vi "Filter Wheel Control.vi"(7 "Calling VI Ref":refnum<vi>) -> ()   [LabVIEW 2020]
uses:
  <vilib>/Utility/miscctls.llb/LVPointTypeDef.ctl
  Hardware Configuration/Hardware Configuration Controls/Device Type.ctl
  Hardware Configuration/Hardware Configuration Controls/Device Function.ctl
  Filter Wheel Type Defs/Filter Wheel Names.ctl
  Device Library/Filter Wheels/FW Type Defs/FW Actions.ctl
panel:
  in  "Tab Control":enum32{"Wheel Control", "Setup"}(tab)
  in  "Filter Wheel":u16(ring) items=["Camera 2 Filter Wheel"]
  in  "Position":T1(radio)
  in  "Pos_Name_06":string
  in  "Pos_Name_07":string
  in  "Pos_Name_08":string
  in  "Pos_Name_09":string
  in  "Pos_Name_10":string
  in  "Filter_Wheel_Name":string
  in  "Pos_Name_01":string
  in  "Pos_Name_02":string
  in  "Pos_Name_03":string
  in  "Pos_Name_04":string
  in  "Pos_Name_05":string
  in  "Filter Wheel Setup":bool=TRUE
  in  "Quit":bool
  # "Filter Wheel Name:"
  # "Position 01 Name:"
  # "Position 06 Name:"
  # "Position 02 Name:"
  # "Position 07 Name:"
  # "Position 03 Name:"
  # "Position 08 Name:"
  # "Position 04 Name:"
  # "Position 09 Name:"
  # "Position 05 Name:"
  # "Position 10 Name:"
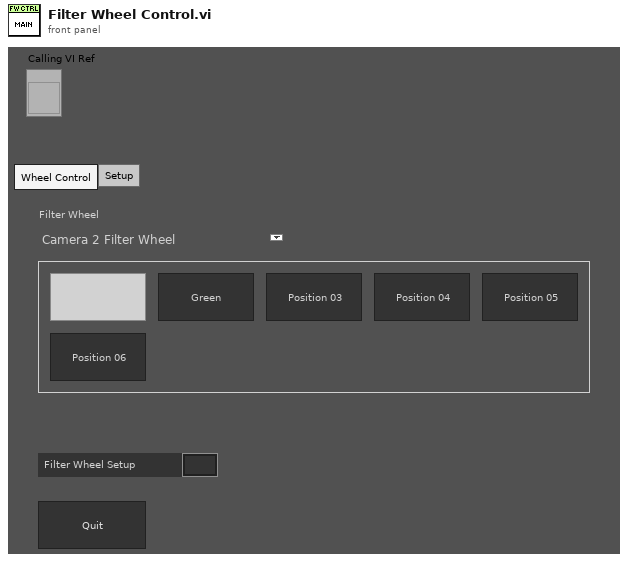
[diagram p1: front panel]
types:
  T1 = enum32{"Pos 01", "Pos 02", "Pos 03", "Pos 04", "Pos 05", "Pos 06", "Pos 07", "Pos 08", "Pos 09", "Pos 10"}
  T2 = typedef "FW Actions.ctl" = enum16{"Set Position", "Get Position", "Get Num Positions", "Set Speed", "Quit"}
  T3 = typedef "Filter Wheel Names.ctl" = string[][]
  T4 = typedef "Device Type.ctl" = enum16{"AOTF", "Camera", "Deformable Mirror", "Laser", "Shutter", "Stage", "Waveform", "FPGA", "Email", "Filter Wheel"}
  T5 = typedef "Device Function.ctl" = enum16{"Primary", "Secondary", "Overview", "Wide Field Drift Correction", "642 nm Excitation", "560 nm Excitation", "940 nm Excitation", "546 nm Excitation", "488 nm Excitation", "405 nm Excitation", "Objective Drift Correction", "4Pi Objective Lock", "Objective XY", "Objective Z", "Sample XY", "Sample Coarse Z", "Sample Z", "4Pi Lower", "4Pi Upper", "Mojo", "Adj Cavity", "Line Scanning", "Alert"}
  T6 = enum16{"Always On", "Always Off", "Off While Running"}
  T7 = typedef "LVPointTypeDef.ctl" = cluster{"Horizontal":i16, "Vertical":i16}
  T8 = enum8{"Enabled", "Disabled", "Disabled and Grayed Out"}
  T9 = typedef "LVRectTypeDef.ctl" = cluster{"Left":i16, "Top":i16, "Right":i16, "Bottom":i16}
  T10 = typedef "LVBoundsTypeDef.ctl" = cluster{"Width":u32, "Height":u32}
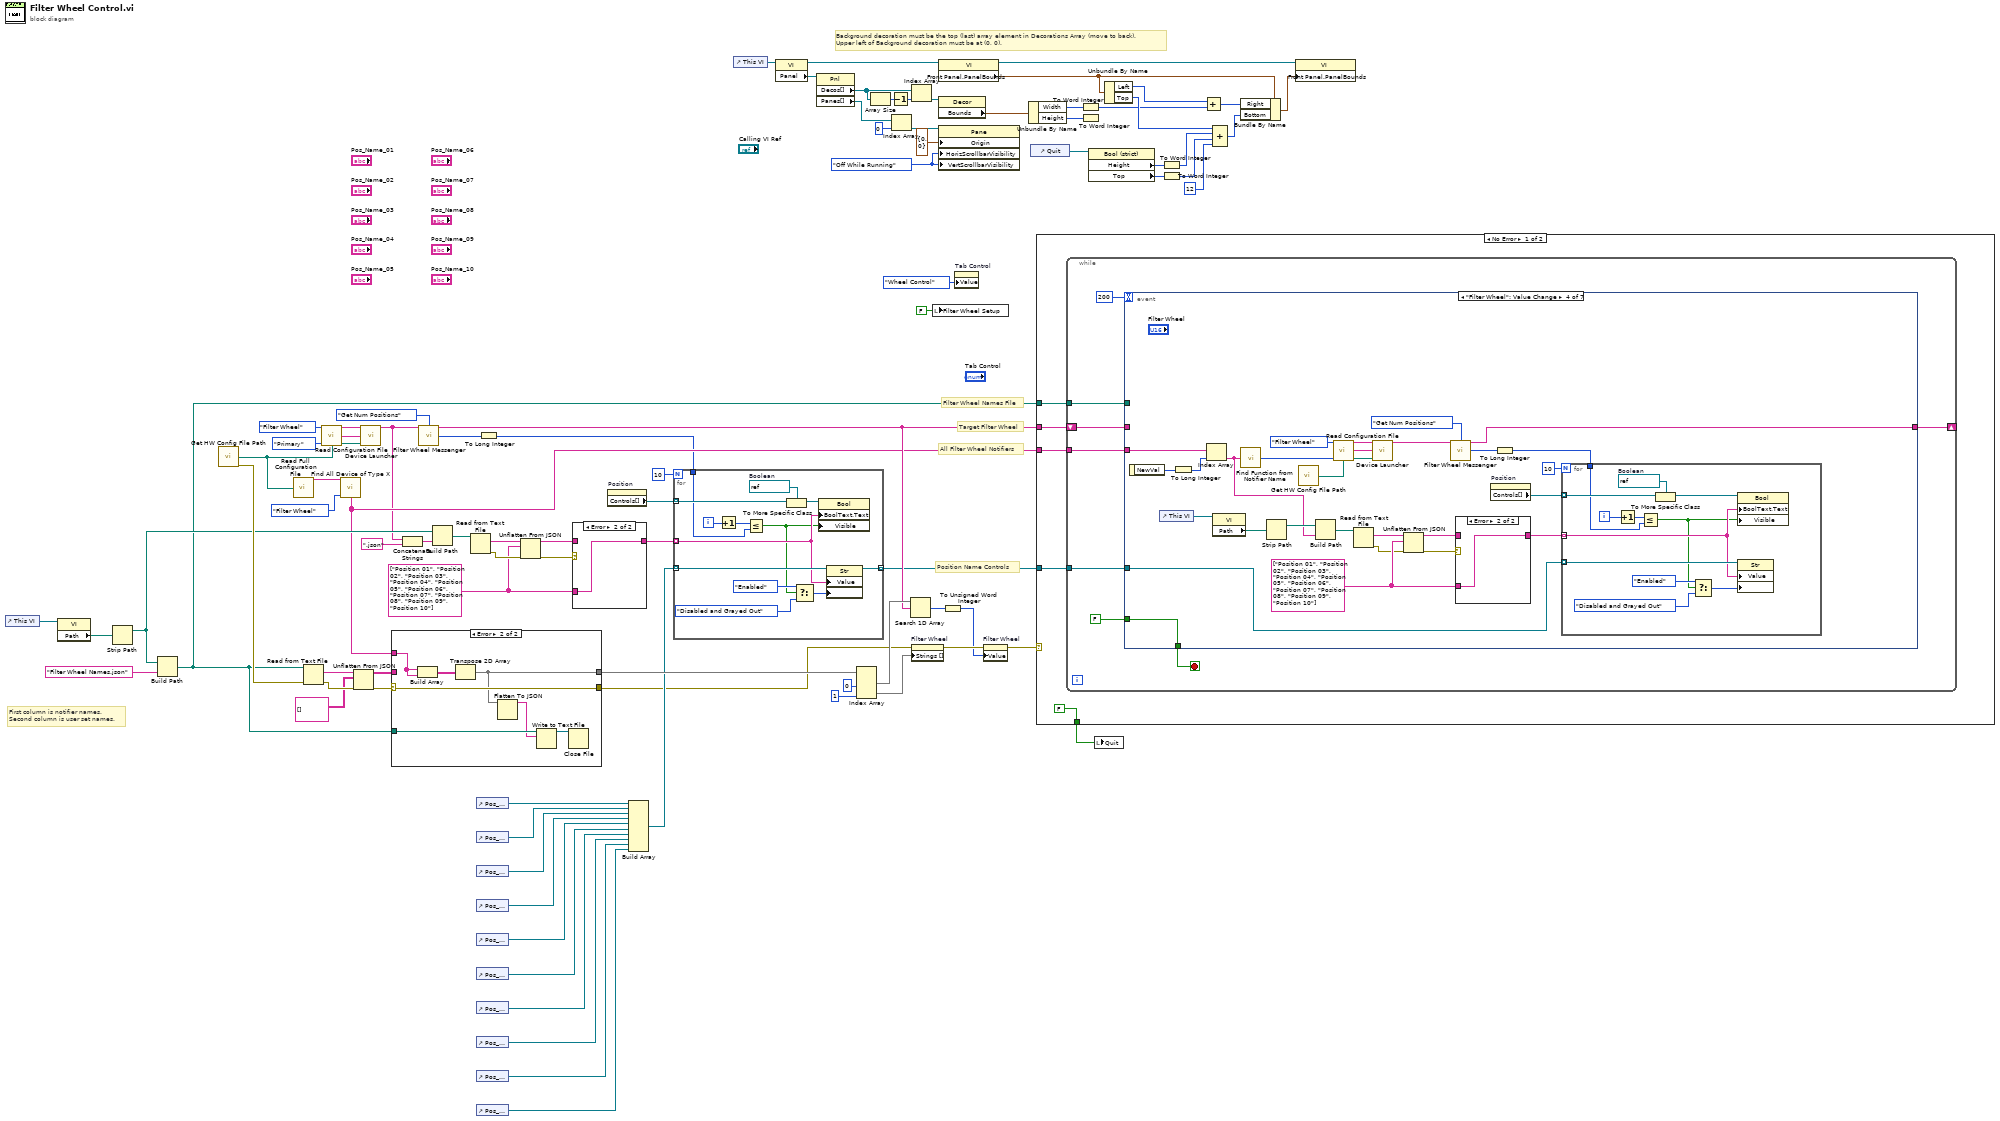
[diagram p0: block diagram]
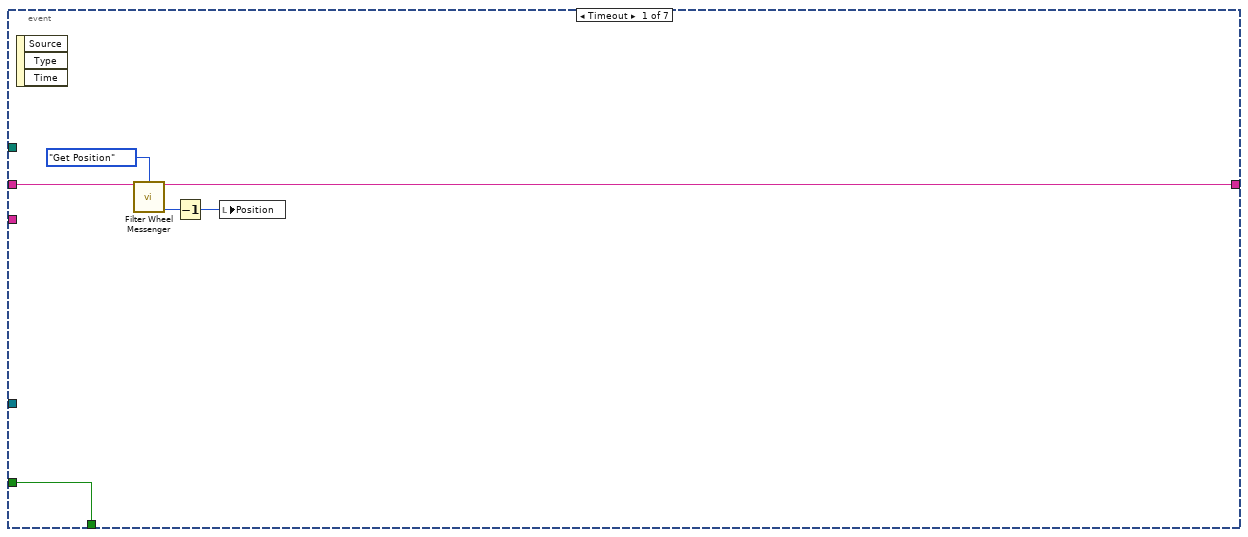
[diagram p2: hidden frame]
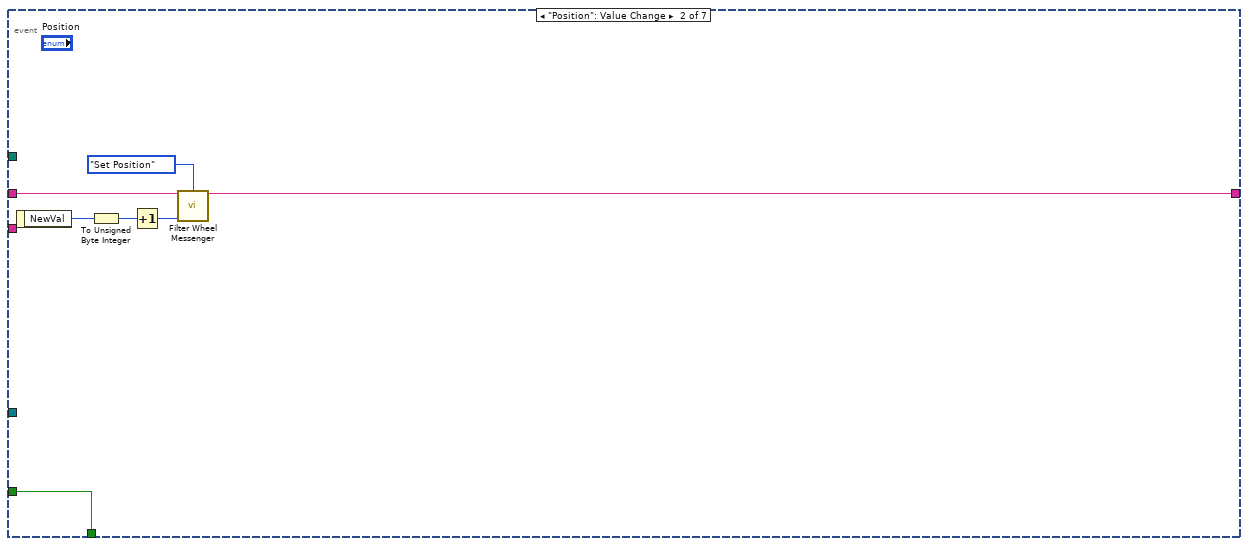
[diagram p3: hidden frame]
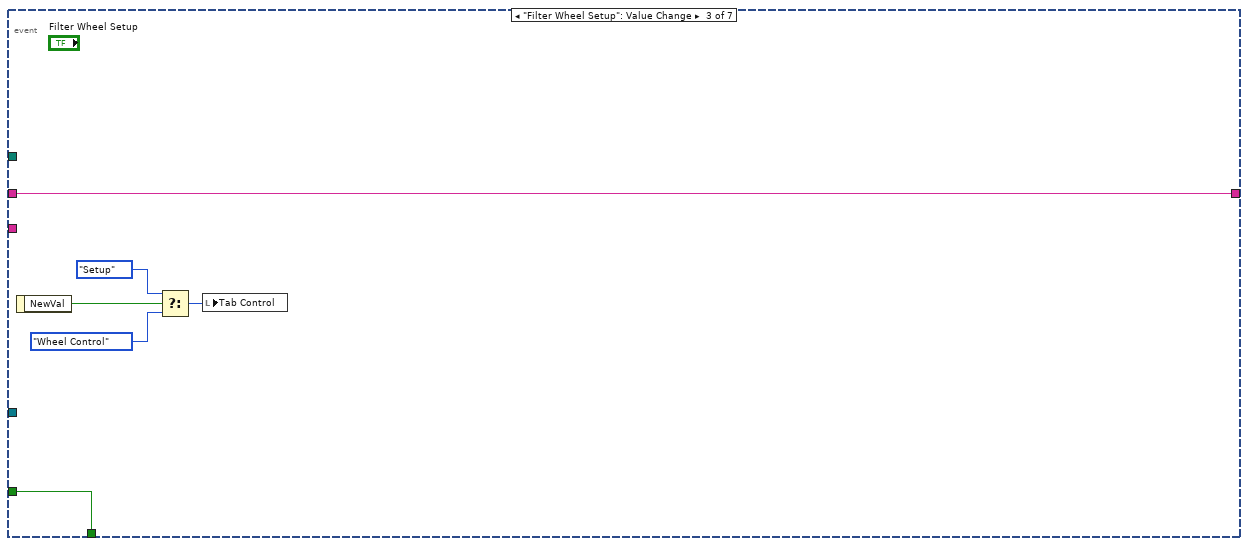
[diagram p4: hidden frame]
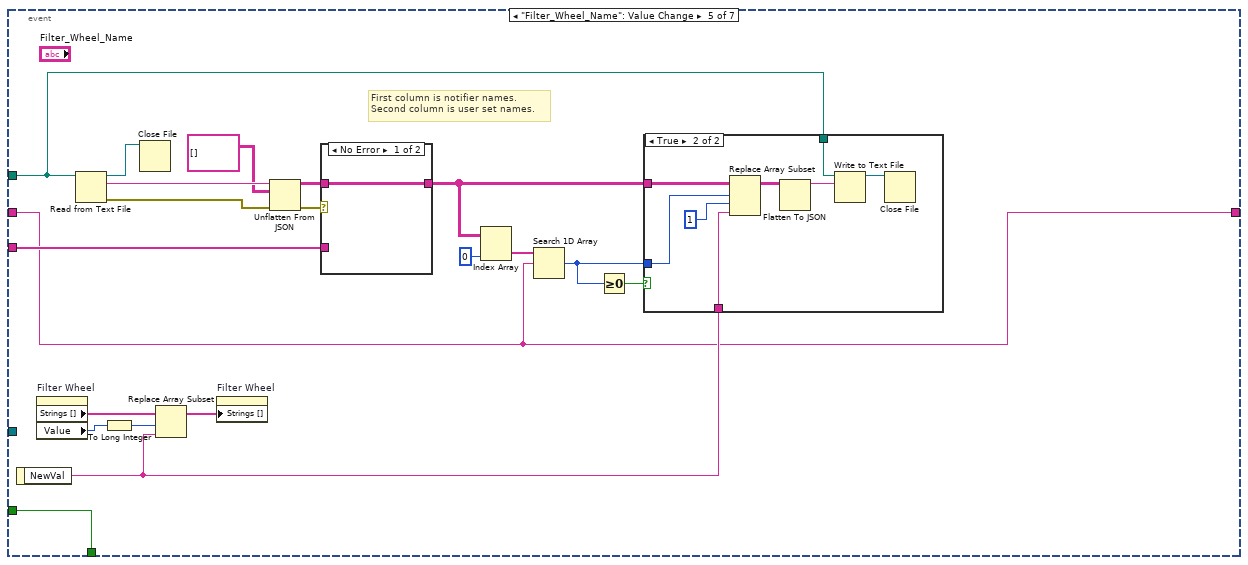
[diagram p6: hidden frame]
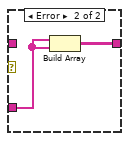
[diagram p8: hidden frame]
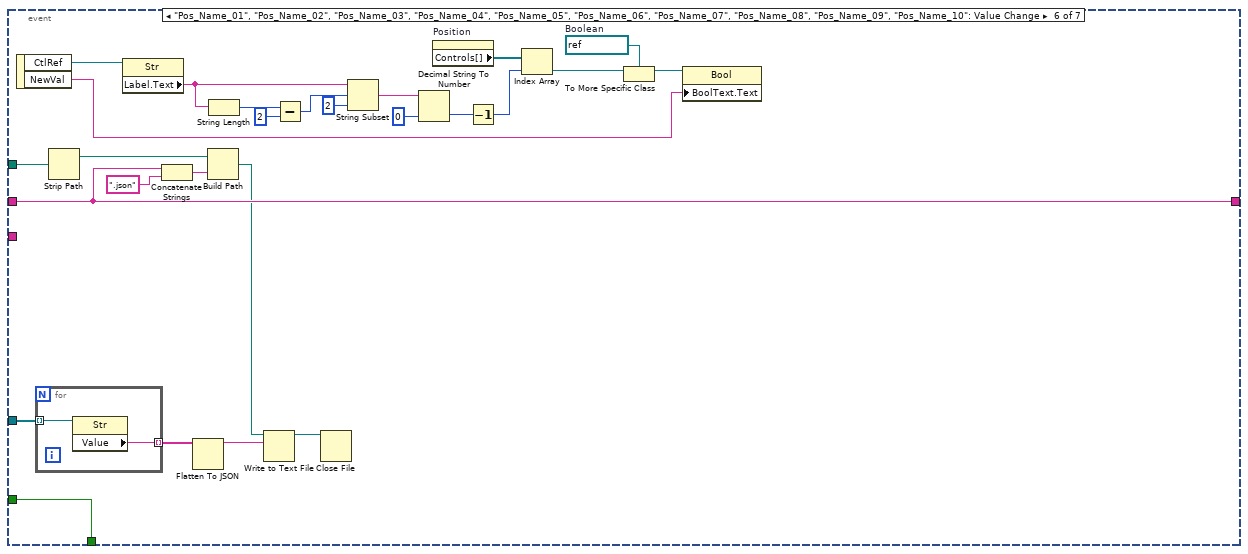
[diagram p9: hidden frame]
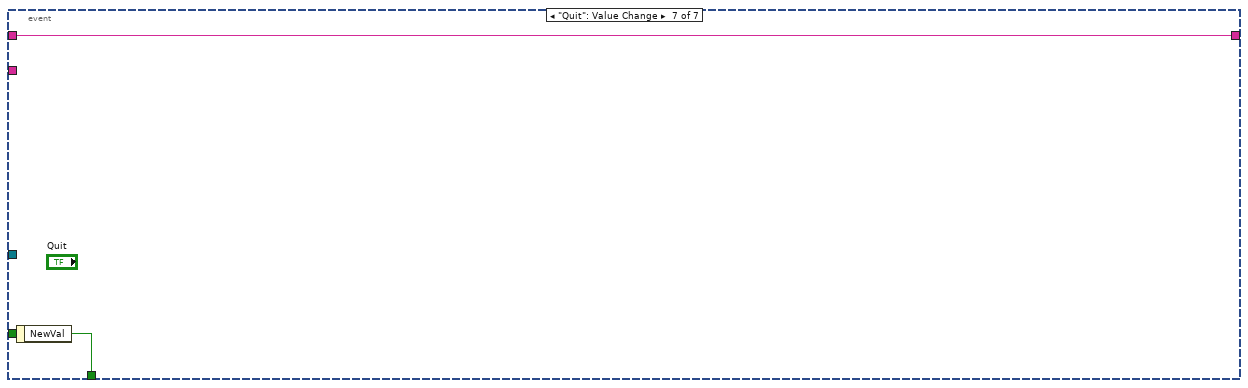
[diagram p10: hidden frame]
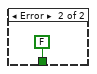
[diagram p11: hidden frame]
diagram:
  w18 = string[] ["Position 01", "Position 02", "Position 03", "Position 04", "Position 05", "Position 06", "Position 07", "Position 08", "Position 09", "Position 10"]
  w73 = T6."Off While Running" ("Vertical Scrollbar Visibility")
  # "Position Name Controls"
  # "All Filter Wheel Notifiers"
  # "Target Filter Wheel"
  # "Filter Wheel Names File"
  # "First column is notifier names.\nSecond column is user set names."
  # "Background decoration must be the top (last) array element in Decorations Array (move to back).\nUpper left of Background decoration must be at (0, 0)."
  n1 = control-ref of="This VI"() -> (w53:refnum<vi>)
  n2 = property class="VI"(reference=w53) -> ("Path"=w52:path)  [unwired: 1 in, 2 out]
  n3 = Strip Path(path=w52) -> (stripped path=w36:path)  [unwired: 1 out]
  n4 = Build Path(base path=w36, name or relative path="Filter Wheel Names.json") -> (appended path=w7:path)
  n5 = call "Get HW Config File Path.vi"() -> ("File Path"=w54:path, "Error"=w37:errorcluster)  [unwired: 14 in]
  n6 = call "Read Full Configuration File.vi"("Config File Path"=w54) -> ("Unique Notifier Names"=w56:string[])  [unwired: 11 in, 3 out]
  n7 = Read from Text File(file (use dialog)=w7, error in=w37) -> (text=w50:string, error out=w49:errorcluster)  [unwired: 2 in, 2 out]
  n8 = call "Read Configuration File.vi"("Device Type"=Device_Type."Filter Wheel", "Device Function"=Device_Function."Primary", "Config File Path"=w54) -> ("Unique Notifier Name"=w61:string, "Device Ports/IDs/Channels"=w59:string[], "Device Engine Path"=w60:path)  [unwired: 9 in, 1 out]
  n9 = call "Find All Device of Type X.vi"("Unique Notifier Names"=w56, "Device Type"=Device_Type."Filter Wheel") -> ("All Devices"=w10:string[])  [unwired: 12 in, 1 out]
  n10 = Unflatten From JSON(JSON string=w50, type and defaults=T3 [] ("Wheel Names"), error in (no error)=w49) -> (value=w46:T3, error out=w47:errorcluster)  [unwired: 4 in]
  n11 = call "Device Launcher.vi"("Notifier Name"=w61, "Device Ports/IDs/Channels"=w59, "Device Engine Path"=w60) -> ("Notifier Name"=w2:string)  [unwired: 11 in, 1 out]
  n12 = case shown="Error" w47 {
    selector: w47 -> [w91 w98]
    tunnel: w46 -> [w92 _]
    tunnel: [w92 w94] -> w45
    tunnel: w10 -> [_ w99]
    tunnel: [w91 w98] -> w12
    tunnel: w7 -> [_ w97]
    frame No Error {
    }
    frame Error {
      n13 = Build Array(w99, w99) -> (w95:string[][])
      n14 = Transpose 2D Array(2D array=w95) -> (transposed array=w94:string[][])
      n15 = Flatten To JSON(anything=w94) -> (JSON string=w93:string)  [unwired: 2 in, 1 out]
      n16 = Write to Text File(file (use dialog)=w97, text=w93) -> (refnum out=w96:refnum<file>)  [unwired: 2 in, 2 out]
      n17 = Close File(refnum=w96) -> ()  [unwired: 1 in, 2 out]
    }
  }
  n18 = Concatenate Strings(w2, ".json" ("string")) -> (w3:string)
  n19 = call "Filter Wheel Messenger.vi"("FW Notifier"=w2, "Actions"=FW_Actions."Get Num Positions") -> ("FW Notifier (Dup)"=w21:string, "Num Positions"=w9:u8)  [unwired: 11 in, 1 out]
  n20 = Build Path(base path=w36, name or relative path=w3) -> (appended path=w33:path)
  n21 = Read from Text File(file (use dialog)=w33) -> (text=w34:string, error out=w35:errorcluster)  [unwired: 3 in, 2 out]
  n22 = control-ref of="Pos_Name_01"() -> (w32:refnum<vi>)
  n23 = control-ref of="Pos_Name_02"() -> (w23:refnum<vi>)
  n24 = control-ref of="Pos_Name_03"() -> (w24:refnum<vi>)
  n25 = control-ref of="Pos_Name_04"() -> (w25:refnum<vi>)
  n26 = control-ref of="Pos_Name_05"() -> (w26:refnum<vi>)
  n27 = control-ref of="Pos_Name_06"() -> (w27:refnum<vi>)
  n28 = control-ref of="Pos_Name_07"() -> (w28:refnum<vi>)
  n29 = control-ref of="Pos_Name_08"() -> (w29:refnum<vi>)
  n30 = control-ref of="Pos_Name_09"() -> (w30:refnum<vi>)
  n31 = control-ref of="Pos_Name_10"() -> (w31:refnum<vi>)
  n32 = To Long Integer(number=w9) -> (32bit integer=w8:i32)
  n33 = Unflatten From JSON(JSON string=w34, type and defaults=w18, error in (no error)=w35) -> (value=w19:string[], error out=w20:errorcluster)  [unwired: 4 in]
  n34 = case shown="Error" w20 {
    tunnel: w19 -> [w100 _]
    tunnel: w18 -> [_ w101]
    tunnel: [w100 w101] -> w16
    frame No Error {
    }
    frame Error {
    }
  }
  n35 = property on="Position" class="RadioBtnsControl (strict)"() -> ("Controls[]"=w13:refnum<vi>[])  [unwired: 2 in, 2 out]
  n36 = Build Array(w32, w23, w24, w25, w26, w27, w28, w29, w30, w31) -> (w15:refnum<vi>[])
  n37 = for {
    N: 10 -> [_]
    tunnel: w16 -> [w109] mode=indexing
    tunnel: w15 -> [w114] mode=indexing
    tunnel: [w113] -> w14 mode=indexing
    tunnel: w13 -> [w112] mode=indexing
    tunnel: w8 -> [w106]
    i -> [w108]
    w111 = refnum<vi> refnum  # Boolean
    n38 = Increment(x=w108) -> (x+1=w107:i32)
    n39 = Less Or Equal?(x=w107, y=w106) -> (x <= y?=w102:bool)
    n40 = To More Specific Class(target class=w111, reference=w112) -> (specific class reference=w110:refnum<vi>)  [unwired: 1 in, 1 out]
    n41 = Select(t=T8."Enabled" ("Disabled"), s=w102, f=T8."Disabled and Grayed Out") -> (s? t:f=w104:T8)
    n42 = property class="Bool"(reference=w110, "BoolText.Text"=w109, "Visible"=w102) -> ()  [unwired: 1 in, 2 out]
    n43 = property class="Str"(reference=w114, "Value"=w109, "DisabledEnum"=w104) -> (reference out=w113:refnum<vi>)  [unwired: 1 in, 1 out]
  }
  n44 = control-ref of="This VI"() -> (w65:refnum<vi>)
  n45 = property class="VI"(reference=w65) -> (reference out=w74:refnum<vi>, "Panel"=w66:refnum<vi>)  [unwired: 1 in, 1 out]
  n46 = property class="Pnl"(reference=w66) -> ("Decos[]"=w64:refnum<vi>[], "Panes[]"=w70:refnum<vi>[])  [unwired: 1 in, 2 out]
  n47 = Index Array(array=w45, index (col) #1=0 ("disabled index (col)"), index (col) #2=1 ("index (col)")) -> (element #1=w38:string[], element #2=w39:string[])  [unwired: 2 in]
  n48 = Array Size(array=w64) -> (size(s)=w62:i32)
  n49 = Decrement(x=w62) -> (x-1=w63:i32)
  n50 = Index Array(array=w70, index=0) -> (element=w69:refnum<vi>)
  n51 = Search 1D Array(1D array=w38, element=w21) -> (index of element=w42:i32)  [unwired: 1 in]
  n52 = property on="Filter Wheel" class="Ring (strict)"(error in=w12, "Strings []"=w39) -> (error out=w43:errorcluster)  [unwired: 1 in, 1 out]
  n53 = Index Array(array=w64, index=w63) -> (element=w72:refnum<vi>)
  n54 = local write "Filter Wheel Setup"(FALSE ("Filter Wheel Setup")) -> ()
  n55 = property class="VI"(reference=w74) -> (reference out=w76:refnum<vi>, "Front Panel.PanelBounds"=w77:T9)  [unwired: 1 in, 1 out]
  n56 = property class="Decor"(reference=w72) -> ("Bounds"=w75:T10)  [unwired: 1 in, 2 out]
  n57 = property class="Pane"(reference=w69, "Origin"=T7 {"Horizontal"=0, "Vertical"=0}, "HorizScrollbarVisibility"=w73, "VertScrollbarVisibility"=w73) -> ()  [unwired: 1 in, 2 out]
  n58 = To Unsigned Word Integer(number=w42) -> (unsigned 16bit integer=w41:u16)
  n59 = property on="Tab Control" class="TabCtl (strict)"("Value"=enum32{"Wheel Control", "Setup"}."Wheel Control" ("Tab Control")) -> ()  [unwired: 2 in, 2 out]
  n60 = property on="Filter Wheel" class="Ring (strict)"(error in=w43, "Value"=w41) -> (error out=w11:errorcluster)  [unwired: 1 in, 1 out]
  n61 = Unbundle By Name(w75) -> ("Width"=w80:u32, "Height"=w83:u32)
  n62 = control-ref of="Quit"() -> (w67:refnum<vi>)
  n63 = case shown="No Error" w11 {
    tunnel: w7 -> [w119 _]
    tunnel: w21 -> [w118 _]
    tunnel: w14 -> [w117 _]
    tunnel: w10 -> [w116 _]
    tunnel: [FALSE FALSE] -> w4
    frame No Error {
      n64 = while {
        shift-right: [w121] -> _
        shift-left: w118 -> [w123]
        tunnel: w119 -> [w125]
        tunnel: w117 -> [w124]
        tunnel: w116 -> [w120]
        stop <- w126 stop-if-true
        n65 = event shown="[3] \"Filter Wheel\": Value Change" {
          selector: _ -> [_ _ _ _ _ _ _]
          dyn-events: _ -> [_ _ _ _ _ _ _]
          timeout: 200 -> [_ _ _ _ _ _ _]
          tunnel: FALSE -> [w133 w140 w146 w175 w209 w246 _]
          tunnel: [w133 w140 w146 w175 w209 w246 w250] -> w126
          tunnel: w125 -> [_ _ _ _ w190 w243 _]
          tunnel: w124 -> [_ _ _ w153 _ w245 _]
          tunnel: w123 -> [w130 w135 w141 _ w192 w240 w249]
          tunnel: [w129 w134 w141 w148 w192 w240 w249] -> w121
          tunnel: w120 -> [_ _ _ w174 w208 _ _]
          event Timeout {
            n66 = event-data() -> ()  [unwired: 1 in, 3 out]
            n67 = call "Filter Wheel Messenger.vi"("FW Notifier"=w130, "Actions"=FW_Actions."Get Position") -> ("FW Notifier (Dup)"=w129:string, "Current Position"=w131:u8)  [unwired: 11 in, 1 out]
            n68 = Decrement(x=w131) -> (x-1=w128:u8)
            n69 = local write "Position"(w128) -> ()
          }
          event "Position": Value Change {
            n70 = event-data() -> ("NewVal"=w139:T1)  [unwired: 1 in]
            n71 = To Unsigned Byte Integer(number=w139) -> (unsigned 8bit integer=w138:u8)
            n72 = Increment(x=w138) -> (x+1=w137:u8)
            n73 = call "Filter Wheel Messenger.vi"("FW Notifier"=w135, "Actions"=FW_Actions."Set Position", "Set Position"=w137) -> ("FW Notifier (Dup)"=w134:string)  [unwired: 10 in, 2 out]
          }
          event "Filter Wheel Setup": Value Change {
            n74 = event-data() -> ("NewVal"=w145:bool)  [unwired: 1 in]
            n75 = Select(t=enum32{"Wheel Control", "Setup"}."Setup" ("Tab Control"), s=w145, f=enum32{"Wheel Control", "Setup"}."Wheel Control" ("Tab Control")) -> (s? t:f=w142:enum32{"Wheel Control", "Setup"})
            n76 = local write "Tab Control"(w142) -> ()
          }
          event "Filter Wheel": Value Change {
            w163 = string[] ["Position 01", "Position 02", "Position 03", "Position 04", "Position 05", "Position 06", "Position 07", "Position 08", "Position 09", "Position 10"]
            n77 = event-data() -> ("NewVal"=w173:u16)  [unwired: 1 in]
            n78 = control-ref of="This VI"() -> (w157:refnum<vi>)
            n79 = To Long Integer(number=w173) -> (32bit integer=w172:i32)
            n80 = Index Array(array=w174, index=w172) -> (element=w154:string)
            n81 = property class="VI"(reference=w157) -> ("Path"=w156:path)  [unwired: 1 in, 2 out]
            n82 = call "Find Function from Notifier Name.vi"("Unique Notifier Name"=w154) -> ("Function"=w167:T5)  [unwired: 14 in]
            n83 = Strip Path(path=w156) -> (stripped path=w155:path)  [unwired: 1 out]
            n84 = call "Get HW Config File Path.vi"() -> ("File Path"=w147:path)  [unwired: 14 in, 1 out]
            n85 = Build Path(base path=w155, name or relative path=w154) -> (appended path=w160:path)
            n86 = call "Read Configuration File.vi"("Device Type"=Device_Type."Filter Wheel", "Device Function"=w167, "Config File Path"=w147) -> ("Unique Notifier Name"=w171:string, "Device Ports/IDs/Channels"=w169:string[], "Device Engine Path"=w170:path)  [unwired: 9 in, 1 out]
            n87 = Read from Text File(file (use dialog)=w160) -> (text=w159:string, error out=w158:errorcluster)  [unwired: 3 in, 2 out]
            n88 = call "Device Launcher.vi"("Notifier Name"=w171, "Device Ports/IDs/Channels"=w169, "Device Engine Path"=w170) -> ("Notifier Name"=w151:string)  [unwired: 11 in, 1 out]
            n89 = Unflatten From JSON(JSON string=w159, type and defaults=w163, error in (no error)=w158) -> (value=w162:string[], error out=w161:errorcluster)  [unwired: 4 in]
            n90 = call "Filter Wheel Messenger.vi"("FW Notifier"=w151, "Actions"=FW_Actions."Get Num Positions") -> ("FW Notifier (Dup)"=w148:string, "Num Positions"=w150:u8)  [unwired: 11 in, 1 out]
            n91 = case shown="Error" w161 {
              tunnel: w162 -> [w188 _]
              tunnel: w163 -> [_ w189]
              tunnel: [w188 w189] -> w165
              frame No Error {
              }
              frame Error {
              }
            }
            n92 = property on="Position" class="RadioBtnsControl (strict)"() -> ("Controls[]"=w166:refnum<vi>[])  [unwired: 2 in, 2 out]
            n93 = To Long Integer(number=w150) -> (32bit integer=w149:i32)
            n94 = for {
              N: 10 -> [_]
              tunnel: w165 -> [w183] mode=indexing
              tunnel: w153 -> [w187] mode=indexing
              tunnel: w166 -> [w186] mode=indexing
              tunnel: w149 -> [w180]
              i -> [w181]
              w185 = refnum<vi> refnum  # Boolean
              n95 = Increment(x=w181) -> (x+1=w182:i32)
              n96 = Less Or Equal?(x=w182, y=w180) -> (x <= y?=w176:bool)
              n97 = To More Specific Class(target class=w185, reference=w186) -> (specific class reference=w184:refnum<vi>)  [unwired: 1 in, 1 out]
              n98 = Select(t=T8."Enabled" ("Disabled"), s=w176, f=T8."Disabled and Grayed Out") -> (s? t:f=w177:T8)
              n99 = property class="Bool"(reference=w184, "BoolText.Text"=w183, "Visible"=w176) -> ()  [unwired: 1 in, 2 out]
              n100 = property class="Str"(reference=w187, "Value"=w183, "DisabledEnum"=w177) -> ()  [unwired: 1 in, 2 out]
            }
          }
          event "Filter_Wheel_Name": Value Change {
            # "First column is notifier names.\nSecond column is user set names."
            n101 = event-data() -> ("NewVal"=w193:string)  [unwired: 1 in]
            n102 = property on="Filter Wheel" class="Ring (strict)"() -> ("Strings []"=w202:string[], "Value"=w201:u16)  [unwired: 2 in, 2 out]
            n103 = Read from Text File(file (use dialog)=w190) -> (refnum out=w191:refnum<file>, text=w207:string, error out=w206:errorcluster)  [unwired: 3 in, 1 out]
            n104 = To Long Integer(number=w201) -> (32bit integer=w200:i32)
            n105 = Close File(refnum=w191) -> ()  [unwired: 1 in, 2 out]
            n106 = Replace Array Subset(array=w202, new element=w193, index=w200) -> (w199:string[])
            n107 = property on="Filter Wheel" class="Ring (strict)"("Strings []"=w199) -> ()  [unwired: 2 in, 2 out]
            n108 = Unflatten From JSON(JSON string=w207, type and defaults=T3 [] ("Wheel Names"), error in (no error)=w206) -> (value=w203:T3, error out=w204:errorcluster)  [unwired: 4 in]
            n109 = case shown="No Error" w204 {
              tunnel: [w218 w219] -> w198
              tunnel: w208 -> [_ w220]
              tunnel: w203 -> [w218 _]
              frame No Error {
              }
              frame Error {
                n110 = Build Array(w220, w220) -> (w219:string[][])
              }
            }
            n111 = Index Array(array=w198, index (col)=0 ("disabled index (col)")) -> (element=w196:string[])  [unwired: 1 in]
            n112 = Search 1D Array(1D array=w196, element=w192) -> (index of element=w194:i32)  [unwired: 1 in]
            n113 = Greater Or Equal To 0?(x=w194) -> (x >= 0?=w195:bool)
            n114 = case shown="True" w195 {
              tunnel: w198 -> [_ w216]
              tunnel: w194 -> [_ w215]
              tunnel: w193 -> [_ w214]
              tunnel: w190 -> [_ w210]
              frame False {
              }
              frame True {
                n115 = Replace Array Subset(array=w216, new element=w214, index (row)=w215, index (col)=1 ("disabled index (col)")) -> (w211:T3)
                n116 = Flatten To JSON(anything=w211) -> (JSON string=w213:string)  [unwired: 2 in, 1 out]
                n117 = Write to Text File(file (use dialog)=w210, text=w213) -> (refnum out=w212:refnum<file>)  [unwired: 2 in, 2 out]
                n118 = Close File(refnum=w212) -> ()  [unwired: 1 in, 2 out]
              }
            }
          }
          event "Pos_Name_01", "Pos_Name_02", "Pos_Name_03", "Pos_Name_04", "Pos_Name_05", "Pos_Name_06", "Pos_Name_07", "Pos_Name_08", "Pos_Name_09", "Pos_Name_10": Value Change {
            w236 = refnum<vi> refnum  # Boolean
            n119 = event-data() -> ("CtlRef"=w235:refnum<vi>, "NewVal"=w223:string)  [unwired: 1 in]
            n120 = for {
              tunnel: w245 -> [w248] mode=indexing
              tunnel: [w247] -> w244 mode=indexing
              n121 = property class="Str"(reference=w248) -> ("Value"=w247:string)  [unwired: 1 in, 2 out]
            }
            n122 = Strip Path(path=w243) -> (stripped path=w242:path)  [unwired: 1 out]
            n123 = property class="Str"(reference=w235) -> ("Label.Text"=w233:string)  [unwired: 1 in, 2 out]
            n124 = Concatenate Strings(w240, ".json" ("string")) -> (w241:string)
            n125 = Flatten To JSON(anything=w244) -> (JSON string=w238:string)  [unwired: 2 in, 1 out]
            n126 = Build Path(base path=w242, name or relative path=w241) -> (appended path=w237:path)
            n127 = String Length(string=w233) -> (length=w232:i32)
            n128 = Write to Text File(file (use dialog)=w237, text=w238) -> (refnum out=w222:refnum<file>)  [unwired: 2 in, 2 out]
            n129 = Subtract(x=w232, y=2) -> (x-y=w230:i32)
            n130 = Close File(refnum=w222) -> ()  [unwired: 1 in, 2 out]
            n131 = String Subset(string=w233, offset (0)=w230, length (rest)=2 ("length (rest)")) -> (substring=w229:string)
            n132 = Decimal String To Number(string=w229, default (0L)=0 ("default (0 I32)")) -> (number=w226:i32)  [unwired: 1 in, 1 out]
            n133 = property on="Position" class="RadioBtnsControl (strict)"() -> ("Controls[]"=w227:refnum<vi>[])  [unwired: 2 in, 2 out]
            n134 = Decrement(x=w226) -> (x-1=w221:i32)
            n135 = Index Array(array=w227, index=w221) -> (element=w225:refnum<vi>)
            n136 = To More Specific Class(target class=w236, reference=w225) -> (specific class reference=w224:refnum<vi>)  [unwired: 1 in, 1 out]
            n137 = property class="Bool"(reference=w224, "BoolText.Text"=w223) -> ()  [unwired: 1 in, 2 out]
          }
          event "Quit": Value Change {
            n138 = event-data() -> ("NewVal"=w250:bool)  [unwired: 1 in]
          }
        }
      }
    }
    frame Error {
    }
  }
  n139 = To Word Integer(number=w80) -> (16bit integer=w82:i16)
  n140 = To Word Integer(number=w83) -> ()  [unwired: 1 out]
  n141 = property class="Bool (strict)"(reference=w67) -> ("Height"=w85:u32, "Top"=w86:i32)  [unwired: 1 in, 2 out]
  n142 = local write "Quit"(w4) -> ()
  n143 = Unbundle By Name(w77) -> ("Left"=w79:i16, "Top"=w90:i16)
  n144 = To Word Integer(number=w85) -> (16bit integer=w88:i16)
  n145 = To Word Integer(number=w86) -> (16bit integer=w89:i16)
  n146 = Add(x=w79, y=w82) -> (x+y=w81:i16)
  n147 = Compound Arithmetic op=ADD(w90, w88, w89, i16 12 ("y")) -> (w84:i16)
  n148 = Bundle By Name(cluster=w77, "Right"=w81, "Bottom"=w84) -> (w78:T9)
  n149 = property class="VI"(reference=w76, "Front Panel.PanelBounds"=w78) -> ()  [unwired: 1 in, 2 out]
